vi "unbundle and rebundle state.vi"(8 "error in (no error)":errorcluster, 9 "state out":refnum<vi>, 10 "state in":refnum<vi>, 11 "TopLevelDiagram in":refnum<vi>) -> (0 "error out":errorcluster)   [LabVIEW 2014, in "CD model script.lvlib"]
uses:
  CD model script.lvlib
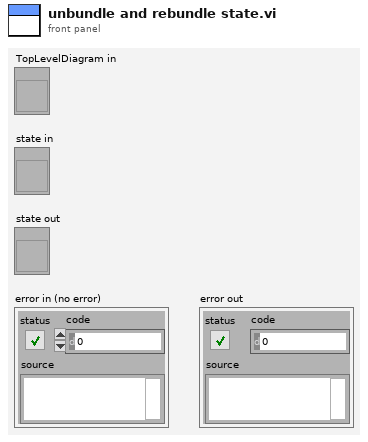
[diagram p1: front panel]
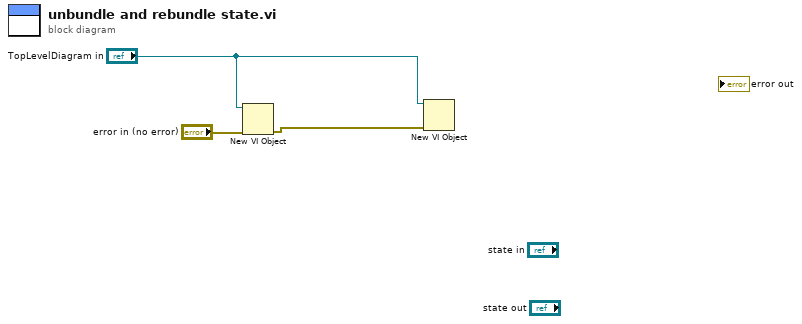
[diagram p0: block diagram]
diagram:
  n1 = New VI Object(owner refnum="TopLevelDiagram in", 8:"error in (no error)") -> (0:w2:errorcluster)  [unwired: 6 in, 1 out]
  n2 = New VI Object(owner refnum="TopLevelDiagram in", 8:w2) -> ()  [unwired: 6 in, 2 out]
